vi "CNTR_SPAN_NPNTS_LMT_CHK.vi"(1 "Center":dbl=10000000.0, 2 "Span":dbl=10000000.0, 3 "Npoints":i32=1, 5 "error in":errorcluster) -> (14 "error out":errorcluster, 15 "Center":dbl=10000000.0, 16 "Span":dbl=10000000.0, 17 "Npoints":i32=1)   [LabVIEW 2018, in "PNA-X.lvlib"]
uses:
  PNA-X.lvlib
panel:
  in  "Limits":T1={"CntrMax"=26500000000.0, "CntrMin"=10000000.0, "SpanMax"=26500000000.0, "SpanMin"=10000000.0, "NptsMax"=16001, "NptsMin"=1}
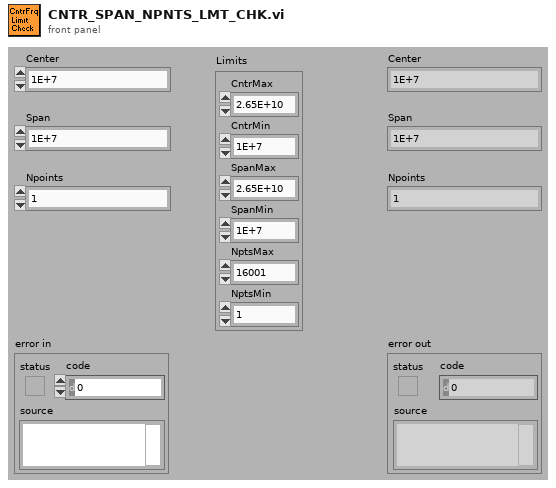
[diagram p1: front panel]
types:
  T1 = cluster{"CntrMax":dbl, "CntrMin":dbl, "SpanMax":dbl, "SpanMin":dbl, "NptsMax":i32, "NptsMin":i32}
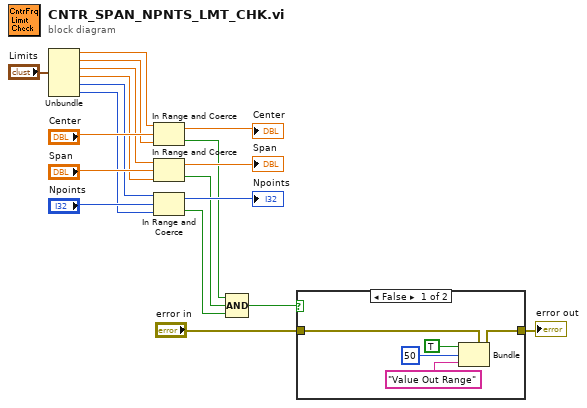
[diagram p0: block diagram]
diagram:
  n1 = Unbundle("Limits") -> ("CntrMax"=w6:dbl, "CntrMin"=w7:dbl, "SpanMax"=w8:dbl, "SpanMin"=w9:dbl, "NptsMax"=w10:i32, "NptsMin"=w11:i32)
  n2 = In Range and Coerce(upper limit=w6, x="Center", lower limit=w7) -> (coerced(x)=→"Center":dbl, In Range?=w5:bool)
  n3 = In Range and Coerce(upper limit=w8, x="Span", lower limit=w9) -> (coerced(x)=→"Span":dbl, In Range?=w4:bool)
  n4 = In Range and Coerce(upper limit=w10, x="Npoints", lower limit=w11) -> (coerced(x)=→"Npoints":i32, In Range?=w3:bool)
  n5 = Compound Arithmetic op=AND(w5, w4, w3) -> (w2:bool)
  n6 = case shown="False" w2 {
    tunnel: "error in" -> [w23 w25]
    tunnel: [w24 w25] -> w19
    frame False {
      n7 = Bundle(cluster=w23, "status"=TRUE, "code"=50, "source"="Value Out Range") -> (w24:errorcluster)
    }
    frame True {
    }
  }
  "error out" <- w19
